vi "pressure monitor.vi"(2 "Data Read Length":u32, 5 "Pressure Monitor Port":refnum<visa-resource-name>, 6 "Command read length":u32, 9 "Separation length":i32) -> (0 "Cold head pressure":string, 1 "pressure":dbl(graph), 3 "Heater Power":string, 4 "power":dbl(graph), 7 "data feedback":string, 8 "command feedback":string)   [LabVIEW 2016]
uses:
  <vilib>/Instr/_visa.llb/VISA Configure Serial Port (Instr).vi
panel:
  out "error out 3":errorcluster
  out "error out 2":errorcluster
  out "error out":errorcluster
  # "configuration"
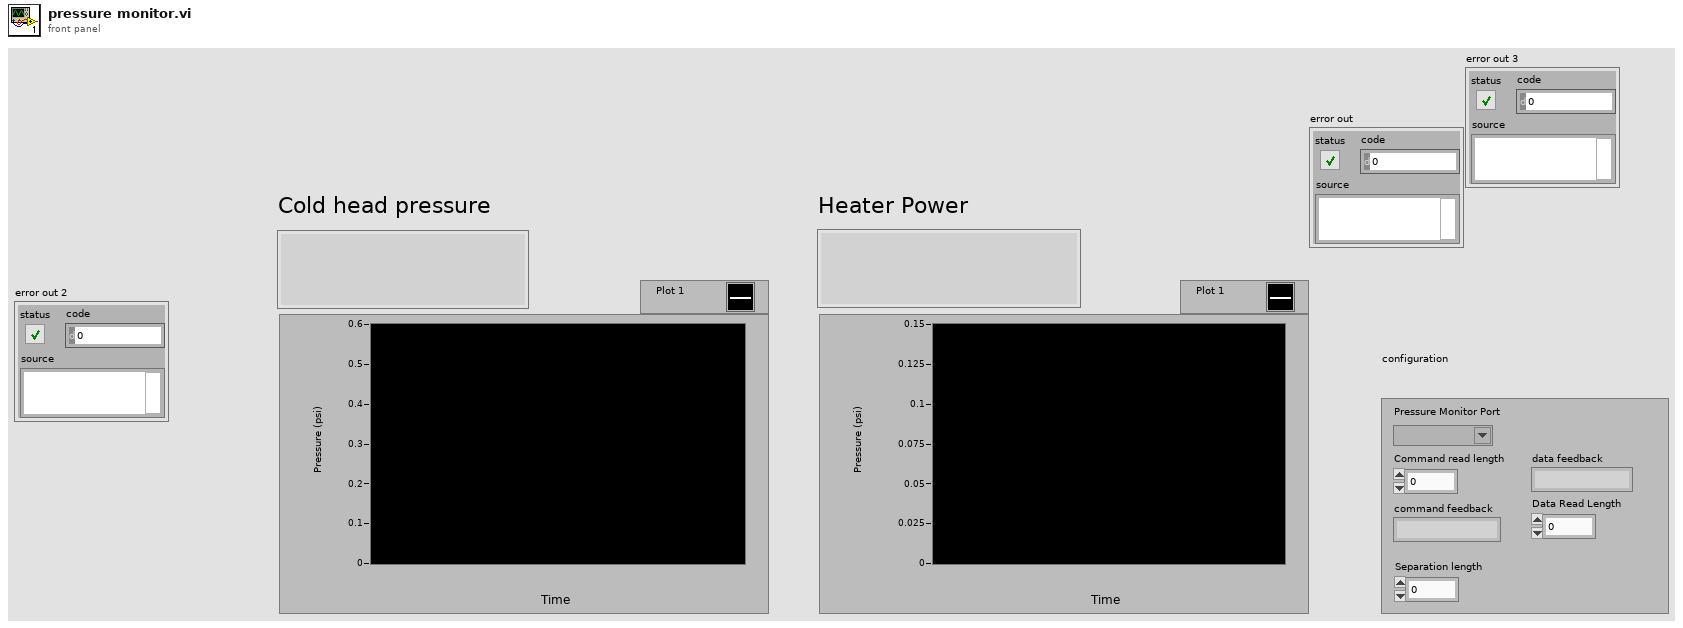
[diagram p1: front panel]
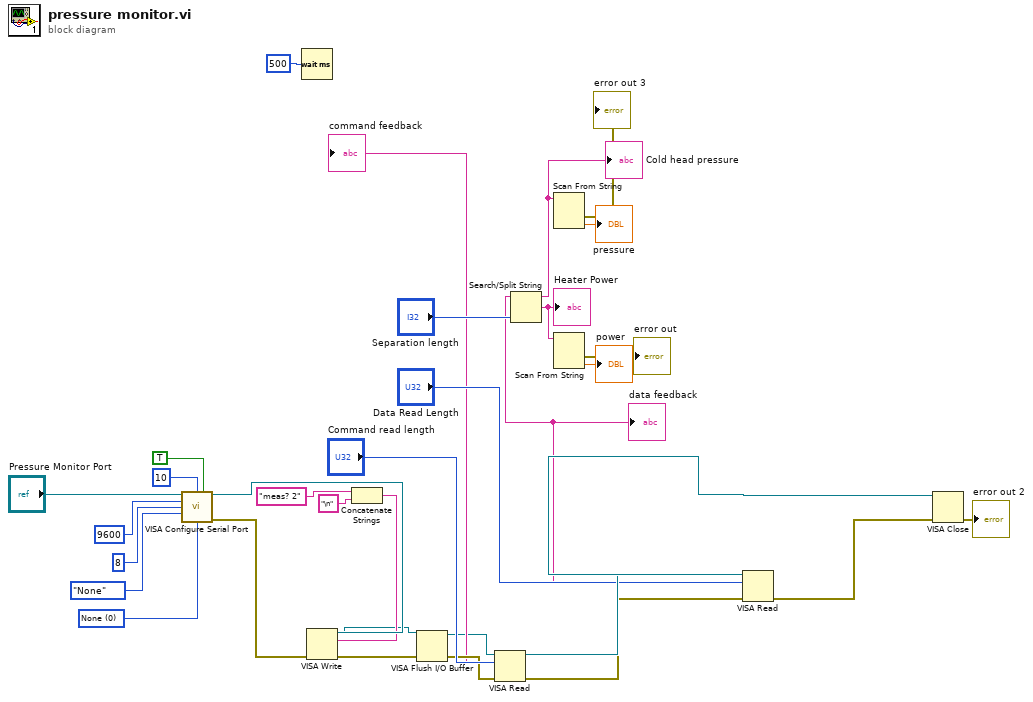
[diagram p0: block diagram]
diagram:
  w24 = u16 0 items=["None", "XON/XOFF", "RTS/CTS", "XON/XOFF & RTS/CTS", "DTR/DSR", "XON/XOFF & DTR/DSR"] ("flow control (0:none)")
  n1 = call-poly "VISA Configure Serial Port"("VISA resource name"="Pressure Monitor Port", "termination char\n(0xA = '\\n' = LF)"=u8 10 ("termination char\n(0xA = '\\n' = LF)"), "Enable Termination\nChar (T)"=TRUE ("Enable Termination\nChar (T)"), "baud rate (9600)"=u32 9600, "data bits (8)"=u16 8, "parity (0:none)"=enum16{"None", "Odd", "Even", "Mark", "Space"}."None", "flow control (0:none)"=w24) -> ("VISA resource name out"=w28:refnum<visa-resource-name>, "error out"=w27:errorcluster)  [unwired: 7 in]
  n2 = Wait (ms)(milliseconds to wait=u32 500) -> ()  [unwired: 1 out]
  n3 = Concatenate Strings("meas? 2" ("string"), "\n" ("string")) -> (w19:string)
  n4 = VISA Write(VISA resource name=w28, write buffer=w19, error in (no error)=w27) -> (VISA resource name out=w5:refnum<visa-resource-name>, error out=w17:errorcluster)  [unwired: 1 out]
  n5 = VISA Flush I/O Buffer(VISA resource name=w5) -> (VISA resource name out=w4:refnum<visa-resource-name>)  [unwired: 2 in, 1 out]
  n6 = VISA Read(VISA resource name=w4, byte count="Command read length", error in (no error)=w17) -> (VISA resource name out=w16:refnum<visa-resource-name>, read buffer=→"command feedback":string, error out=w15:errorcluster)  [unwired: 1 out]
  n7 = VISA Read(VISA resource name=w16, byte count="Data Read Length", error in (no error)=w15) -> (VISA resource name out=w23:refnum<visa-resource-name>, read buffer=w7:string, error out=w22:errorcluster)  [unwired: 1 out]
  "data feedback" <- w7
  n8 = Search/Split String(string=w7, offset (0)="Separation length") -> (substring before match=w12:string, match + rest of string=w11:string)  [unwired: 1 in, 1 out]
  "Cold head pressure" <- w12
  "Heater Power" <- w11
  n9 = Scan From String(input string=w12) -> (error out=→"error out 3":errorcluster, output 1=→"pressure":dbl)  [unwired: 4 in, 2 out]
  n10 = Scan From String(input string=w11) -> (error out=→"error out":errorcluster, output 1=→"power":dbl)  [unwired: 4 in, 2 out]
  n11 = VISA Close(VISA resource name=w23, error in (no error)=w22) -> (error out=→"error out 2":errorcluster)
